vi "1.4.4-Lidar Motor Encoder.vi"   [LabVIEW 2010]
uses:
  <vilib>/eio/EIONode/EIONode.xnode
  <vilib>/rvi/eio/nirviEIOImplementation/nirviEIOImplementation.xnode
  <vilib>/rvi/eio/common/nirviEmuClasses.ctl
  1.0-Hindbrain Global.vi
  <vilib>/rvi/eio/common/nirviEmuTemplateMethod_noerrors.vi
types:
  T1 = typedef "nirviEmuClasses.ctl" = enum16{"IO Read", "IO Write", "Method", "Property Read", "Property Write"}
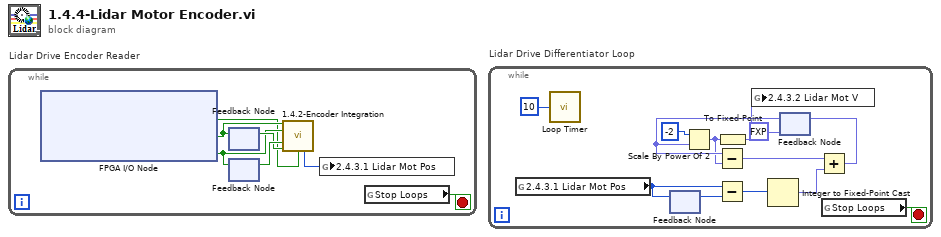
[diagram p0: block diagram]
diagram:
  n1 = while "Lidar Drive Encoder Reader" {
    stop <- w7 stop-if-true
    n2 = xnode "FPGA I/O Node"() -> ("Lidar Drive Encoder Index"=w2:bool, "Lidar Drive Encoder B"=w3:bool, "Lidar Drive Encoder A"=w4:bool)  [unwired: 3 in, 3 out]
    n3 = feedback #1() -> (w5:bool)  [unwired: 1 in]
    n4 = feedback-in #1(w3) -> ()
    n5 = feedback-in #2(w4) -> ()
    n6 = feedback #2() -> (w6:bool)  [unwired: 1 in]
    n7 = call "1.4.2-Encoder Integration.vi"("Encoder B"=w3, "Encoder A"=w4, "Encoder A Old"=w6, "Encoder B Old"=w5, "Encoder Index"=w2) -> ("Current count"=w1:i32)  [unwired: 5 in, 5 out]
    n8 = global write "1.0-Hindbrain Global.vi" "2.4.3.1 Lidar Mot Pos"(w1) -> ()
    n9 = global read "1.0-Hindbrain Global.vi" "Stop Loops"() -> (w7:bool)
  }
  n10 = while "Lidar Drive Differentiator Loop" {
    stop <- w76 stop-if-true
    n11 = global read "1.0-Hindbrain Global.vi" "2.4.3.1 Lidar Mot Pos"() -> (w75:i32)
    n12 = call "Loop Timer"("Count(mSec)"=u32 10 ("Count(Ticks)")) -> ()  [unwired: 1 out]
    n13 = feedback #3() -> (w74:i32)  [unwired: 1 in]
    n14 = feedback-in #3(w75) -> ()
    n15 = Subtract(x=w75, y=w74) -> (x-y=w73:i32)
    n16 = Integer to Fixed-Point Cast(integer=w73) -> (fixed-point=w67:fxp<+/-,12,10>)  [unwired: 1 in]
    n17 = feedback #4(fxp<+/-,12,10> 0.0) -> (w69:fxp<+/-,12,10>)
    n18 = Scale By Power Of 2(n=i8 -2, x=w69) -> (x*2^n=w66:fxp<+/-,12,10>)
    n19 = Subtract(x=w69, y=w66) -> (x-y=w72:fxp<+/-,12,10>)
    n20 = To Fixed-Point(number=w66) -> (fixed-point=w65:fxp<+/-,10,8>)  [unwired: 1 in]
    n21 = global write "1.0-Hindbrain Global.vi" "2.4.3.2 Lidar Mot V"(w65) -> ()
    n22 = Add(x=w72, y=w67) -> (x+y=w68:fxp<+/-,12,10>)
    n23 = feedback-in #4(w68) -> ()
    n24 = global read "1.0-Hindbrain Global.vi" "Stop Loops"() -> (w76:bool)
  }
